vi "Find Pressure and Tangents.vi"(11 "XYGraph in":refnum<vi>) -> (2 "Tangents":dbl[][](array[numeric]), 3 "Pressure":dbl)   [LabVIEW 2013, in "main.lvlib"]
uses:
  main.lvlib
  Controls/Enum Globals.ctl
  Controls/Enum Variables.ctl
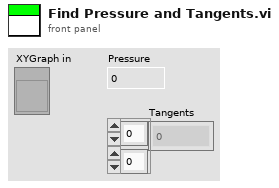
[diagram p1: front panel]
types:
  T1 = typedef "main.lvlib/Enum Variables.ctl" = enum16{"SetAcqFilter", "GetAcqFilter", "Set Filter", "Get Filter", "Set Height", "Get Height", "Set Blue Pressure", "Get Blue Pressure", "Set Red Pressure", "Get Red Pressure", "Init", "Reset Pressure", "Set Red Cursors", "Get Red Cursors", "Set Blue Cursors", "Get Blue Cursors", "Set Language", "Get Language", "Set Active Graphs", "Get ActiveGraphs", "Set Method", "Get Method", "Set Encryption", "Get Encryption", "Set ExcelVersion", "Get ExcelVersion", "Set DICOM Avail", "Get DICOM Avail", "Set DICOM Encode", "Get DICOM Encode", "Set JournalExport", "Get JournalExport", "Set Sequence", "Get Sequence", "Set DAQ Connected", "Get DAQ Connected", "Set Current Graph", "Get Current Graph", "Set General Settings", "Get Hyphenation", "Set Arm Calc Method", "Get Arm Calc Method", "Set Dicom Tags", "Get Dicom Tags", "Set BT Serial", "Get BT Serial", "Set BT Accepted Serials", "Get BT Accepted Serials", "Get BT License", "Set BT License"}
  T2 = typedef "main.lvlib/Enum Globals.ctl" = enum16{"Init", "Set DataPath", "Set Freq", "Get"}
  T3 = typedef "LVCursorListTypeDef.ctl" = cluster{"Name":string, "Color":u32, "Style":u8, "Point Style":u8, "Name Visible":bool, "Allow Drag":bool, "Cursor Mode":u32, "Plot":i32, "Index":i32, "Position":cluster{"X":dbl, "Y":dbl}, "X Scale":u32, "Y Scale":u32, "Watch Plots":i32[], "Watch All Plots":bool, "Plot Area":i32, "Label Offset":cluster{"X":dbl, "Y":dbl}}[]
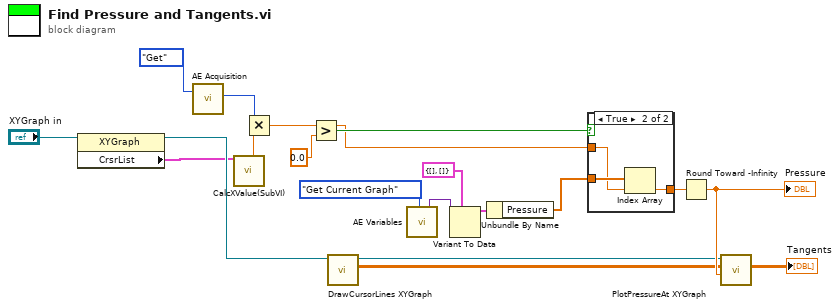
[diagram p0: block diagram]
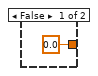
[diagram p2: hidden frame]
diagram:
  n1 = property class="XYGraph"(reference="XYGraph in") -> (reference out=w14:refnum<vi>, "CrsrList"=w11:T3)  [unwired: 1 in, 1 out]
  n2 = call "AE Acquisition.vi"("Action"=Enum_Globals."Get") -> ("Freq Out"=w13:i32)  [unwired: 7 in, 3 out]
  n3 = call "CalcXValue(SubVI).vi"("CrsrList"=w11) -> ("X-value"=w12:dbl)  [unwired: 8 in, 2 out]
  n4 = Multiply(x=w13, y=w12) -> (x*y=w2:dbl)
  n5 = Greater?(x=w2, y=0.0) -> (0:w4:bool)
  n6 = call "DrawCursorLines XYGraph.vi"("CtlRef"=w14) -> ("Array"=w8:dbl[][], "reference out"=w7:refnum<vi>)  [unwired: 9 in]
  n7 = call "AE Variables.vi"("Action"=Enum_Variables."Get Current Graph") -> ("Variant"=w16:variant)  [unwired: 11 in, 7 out]
  n8 = Variant To Data(type=cluster{"Pressure":dbl[], "Graph":dbl[]} {"Pressure"=[], "Graph"=[]}, Variant=w16) -> (data=w18:cluster{"Pressure":dbl[], "Graph":dbl[]})  [unwired: 1 in, 1 out]
  n9 = Unbundle By Name(w18) -> ("Pressure"=w19:dbl[])
  n10 = case shown="True" w4 {
    tunnel: w19 -> [_ w23]
    tunnel: w2 -> [_ w22]
    tunnel: [0.0 w21] -> w1
    frame False {
    }
    frame True {
      n11 = Index Array(array=w23, index=w22) -> (element=w21:dbl)
    }
  }
  n12 = Round Toward -Infinity(1:w1) -> (0:w10:dbl)
  "Pressure" <- w10
  n13 = call "PlotPressureAt XYGraph.vi"("Press In"=w10, "Array"=w8, "reference"=w7) -> ("Array Out"=→"Tangents":dbl[][])  [unwired: 8 in]
